vi "Set control.vi"(0 "BMC in":refnum<class "BMC.lvclass">, 1 "CIUsbLib.IHostDrv":refnum<k7>, 2 "CIUSBLib_SetControl":T1(ring), 3 "error in (no error)":errorcluster) -> (7 "BMC out":refnum<class "BMC.lvclass">, 8 "CiUsbLib.IHostDrv":refnum<k7>, 10 "error out":errorcluster)   [LabVIEW 2012, in "BMC.lvclass"]
uses:
  BMC.lvclass
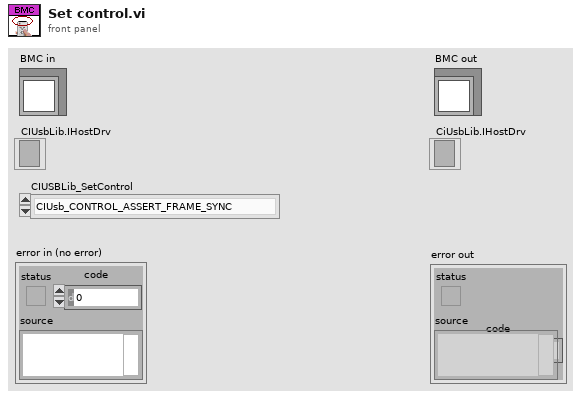
[diagram p1: front panel]
types:
  T1 = enum16{"CIUsb_CONTROL_ASSERT_FRAME_SYNC", "CIUsb_CONTROL_DEASSERT_FRAME_SYNC", "CIUsb_CONTROL_ASSERT_FRESET", "CIUsb_CONTROL_DEASSERT_FRESET", "CIUsb_CONTROL_ASSERT_HV_ENAB", "CIUsb_CONTROL_DEASSERT_HV_ENAB", "CIUsb_CONTROL_ASSERT_LV_SHDN", "CIUsb_CONTROL_DEASSERT_LV_SHDN", "CIUsb_CONTROL_ASSERT_EXT_I2C", "CIUsb_CONTROL_DEASSERT_EXT_I2C", "CIUsb_CONTROL_MINI_MODE"}
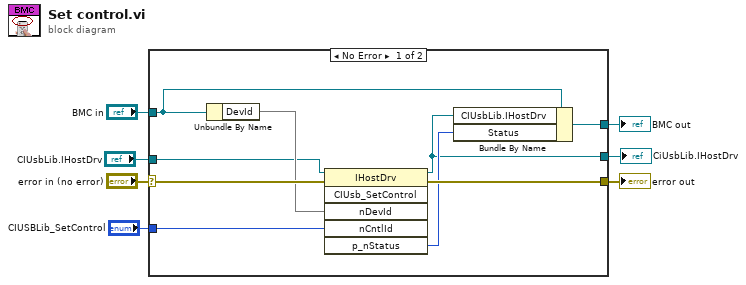
[diagram p0: block diagram]
diagram:
  n1 = case shown="No Error" "error in (no error)" {
    selector: "error in (no error)" -> [w15 w18]
    tunnel: [w16 w18] -> w6
    tunnel: [w13 w17] -> w4
    tunnel: "BMC in" -> [w14 w17]
    tunnel: [w10 _] -> w3
    tunnel: "CIUSBLib_SetControl" -> [w9 _]
    tunnel: "CIUsbLib.IHostDrv" -> [w8 _]
    frame No Error {
      n2 = Unbundle By Name(w14) -> ("DevId"=w12)
      n3 = invoke class="IHostDrv" method="CIUsb_SetControl"(reference=w8, error in=w15, "nDevId"=w12, "nCntlId"=w9) -> (reference out=w10:refnum<k7>, error out=w16:errorcluster, "p_nStatus"=w11:i32)  [unwired: 2 in, 3 out]
      n4 = Bundle By Name(cluster=w14, "CIUsbLib.IHostDrv"=w10, "Status"=w11) -> (w13:refnum<class "BMC.lvclass">)
    }
    frame Error {
    }
  }
  "error out" <- w6
  "BMC out" <- w4
  "CiUsbLib.IHostDrv" <- w3
